vi "Reload.vi"(0 "Display State In":T1, 9 "Container State":T2, 11 "error in (no error)":errorcluster) -> (4 "Display State Out":T1, 15 "error out":errorcluster)   [LabVIEW 2020, in "WebView2 Control.xctl"]
uses:
  WebView2 Control.xctl
  <vilib>/_xctls/Container State.ctl
  State.ctl
  Webview2 Lib/WebView2 Control Object/WebView2 Control.lvclass
  <vilib>/_xctls/XControlSupport.lvlib
panel:
  # "Add Controls & Indicators that form the parameters of the method here. Hook them to the connector pane. Do not delete the controls & indicators that are already hooked to the connector pane.\n \nTo setup the parameters  for this method, right click on this item in the Project Tree & select \"Configure Method...\"."
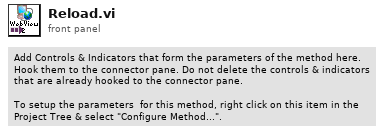
[diagram p1: front panel]
types:
  T1 = typedef "WebView2 Control.xctl/State.ctl" = cluster{"Control Object Ref":refnum<data-value>}
  T2 = typedef "XControlSupport.lvlib/Container State.ctl" = cluster{"Indicator?":bool, "Run Mode?":bool, " Refnum":refnum<vi>}
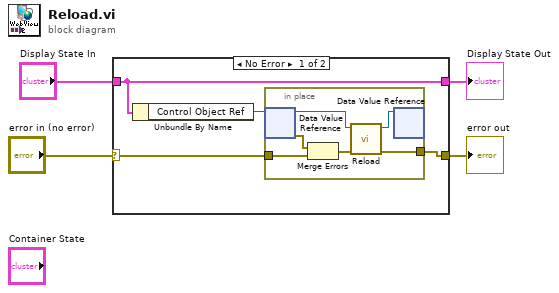
[diagram p0: block diagram]
diagram:
  n1 = case shown="No Error" "error in (no error)" {
    selector: "error in (no error)" -> [w5 w16]
    tunnel: [w6 w16] -> w4
    tunnel: "Display State In" -> [w8 w15]
    tunnel: [w8 w15] -> w1
    frame No Error {
      n2 = Unbundle By Name(w8) -> ("Control Object Ref"=w7:refnum<data-value>)
      n3 = in-place {
        in-place-border: [w11] -> w6
        in-place-border: w5 -> [w9]
        n4 = in-place-dvr #1(w7) -> (w14:refnum<class "WebView2 Control.lvclass">, w12:errorcluster)
        n5 = Merge Errors(w12, w9) -> (w10:errorcluster)
        n6 = call "Reload.vi"("error in (no error)"=w10, "WebView2 Control in"=w14) -> ("error out"=w11:errorcluster, "WebView2 Control out"=w13:refnum<class "WebView2 Control.lvclass">)  [unwired: 8 in]
        n7 = in-place-dvr #1(w13) -> ()  [unwired: 2 out]
      }
    }
    frame Error {
    }
  }
  "Display State Out" <- w1
  "error out" <- w4
